vi "quadrant-photodiode-subvi.vi"(0 "Mode":enum16{"Start", "Read", "End"}(ring), 5 "Display":bool=TRUE, 7 "Handle":i32, 9 "Averages":i32=1 min=1) -> (4 "coerced(x)":dbl, 6 "coerced(y)":dbl, 8 "Power (mw)":dbl)   [LabVIEW 2014]
uses:
  Globals/tirf-lock-globals.vi
  Program Files/Mad City Labs/TIRF-Lock/LabView 32-bit/TIRF-Lock.dll
panel:
  out "coerced(sum)":dbl
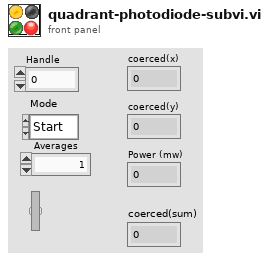
[diagram p1: front panel]
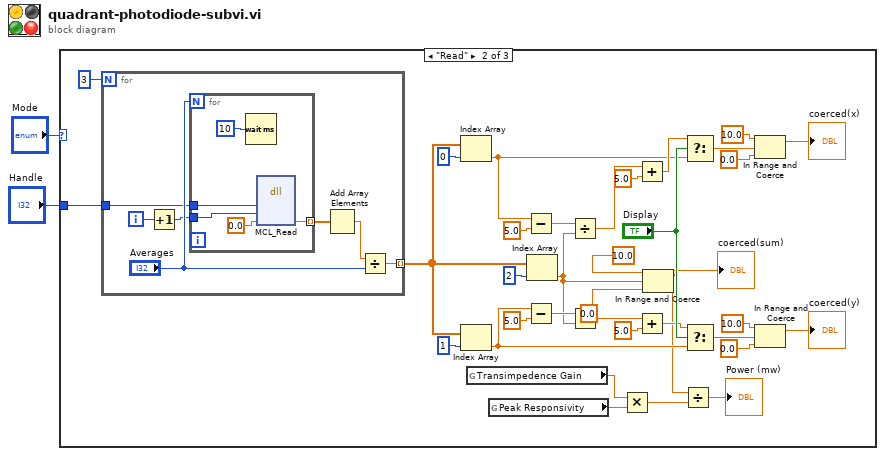
[diagram p0: block diagram]
diagram:
  n1 = case shown="\"Read\"" "Mode" {
    tunnel: "Handle" -> [_ w37 _]
    frame "Start", Default {
    }
    frame "Read" {
      n2 = for {
        N: 3 -> [_]
        tunnel: [w41] -> w35 mode=indexing
        tunnel: w37 -> [w38]
        i -> [w39]
        n3 = Increment(x=w39) -> (x+1=w40:i32)
        n4 = for {
          N: "Averages" -> [_]
          tunnel: w38 -> [w46]
          tunnel: [w48] -> w43 mode=indexing
          tunnel: w40 -> [w47]
          n5 = Wait (ms)(milliseconds to wait=10) -> ()  [unwired: 1 out]
          n6 = dll-call lib="C:/Program Files/Mad City Labs/TIRF-Lock/LabView 32-bit/TIRF-Lock.dll" fn="MCL_Read" label="tirf read"("handle"=w46, "axis"=w47, "readValue"=0.0) -> ("readValue"=w48:dbl)  [unwired: 5 in, 3 out]
        }
        n7 = Add Array Elements(numeric array=w43) -> (sum=w44:dbl)
        n8 = Divide(x=w44, y="Averages") -> (x/y=w41:dbl)
      }
      n9 = Index Array(array=w35, index=0) -> (element=w22:dbl)
      n10 = Index Array(array=w35, index=1) -> (element=w20:dbl)
      n11 = global read "tirf-lock-globals.vi" "Transimpedence Gain"() -> (w7:dbl)
      n12 = global read "tirf-lock-globals.vi" "Peak Responsivity"() -> (w6:dbl)
      n13 = Subtract(x=w22, y=5.0) -> (x-y=w30:dbl)
      n14 = Subtract(x=w20, y=5.0) -> (x-y=w26:dbl)
      n15 = Index Array(array=w35, index=2) -> (element=w9:dbl)
      n16 = Divide(x=w30, y=w9) -> (x/y=w29:dbl)
      n17 = Divide(x=w26, y=w9) -> (x/y=w25:dbl)
      n18 = Multiply(x=w7, y=w6) -> (x*y=w5:dbl)
      n19 = Add(x=w29, y=5.0) -> (x+y=w23:dbl)
      n20 = Add(x=w25, y=5.0) -> (x+y=w21:dbl)
      n21 = In Range and Coerce(upper limit=10.0, x=w9, lower limit=0.0) -> (coerced(x)=w8:dbl)  [unwired: 1 out]
      "coerced(sum)" <- w8
      n22 = Divide(x=w8, y=w5) -> (x/y=→"Power (mw)":dbl)
      n23 = Select(t=w23, s="Display", f=w22) -> (s? t:f=w17:dbl)
      n24 = Select(t=w21, s="Display", f=w20) -> (s? t:f=w14:dbl)
      n25 = In Range and Coerce(upper limit=10.0, x=w17, lower limit=0.0) -> (coerced(x)=→"coerced(x)":dbl)  [unwired: 1 out]
      n26 = In Range and Coerce(upper limit=10.0, x=w14, lower limit=0.0) -> (coerced(x)=→"coerced(y)":dbl)  [unwired: 1 out]
    }
    frame "End" {
    }
  }
